vi "Factory Create.vi"(8 "Error In":errorcluster, 10 "IConfigure":refnum<class "IConfigure.lvclass">, 11 "reference in":refnum<class "Scope Simulated.lvclass">) -> (0 "Error Out":errorcluster, 3 "reference out":refnum<class "Scope Simulated.lvclass">)   [LabVIEW 2023, in "Scope Simulated.lvlib" / "Scope Simulated.lvclass"]
uses:
  Scope Simulated.lvclass
  Scope Simulated.lvclass/Scope Simulated.ctl
  Interfaces/IConfigure/IConfigure.lvclass
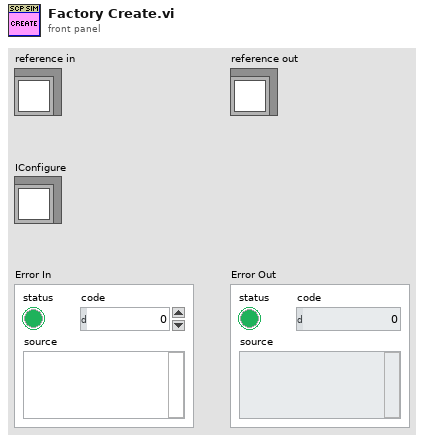
[diagram p1: front panel]
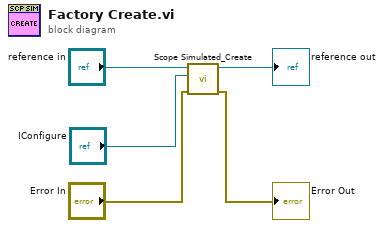
[diagram p0: block diagram]
diagram:
  n1 = call "Scope Simulated_Create.vi"("Error In"="Error In", "IConfigure"="IConfigure", "reference in"="reference in") -> ("Error Out"=→"Error Out":errorcluster, "reference out"=→"reference out":refnum<class "Scope Simulated.lvclass">)  [unwired: 7 in]
